vi "fly.vi"(8 "error in (no error)":errorcluster, 11 "FlyWithWings in":refnum<class "FlyWithWings.lvclass">) -> (0 "error out":errorcluster, 2 "String":string, 3 "FlyWithWings out":refnum<class "FlyWithWings.lvclass">)   [LabVIEW 2013, in "FlyWithWings.lvclass"]
uses:
  FlyWithWings.lvclass
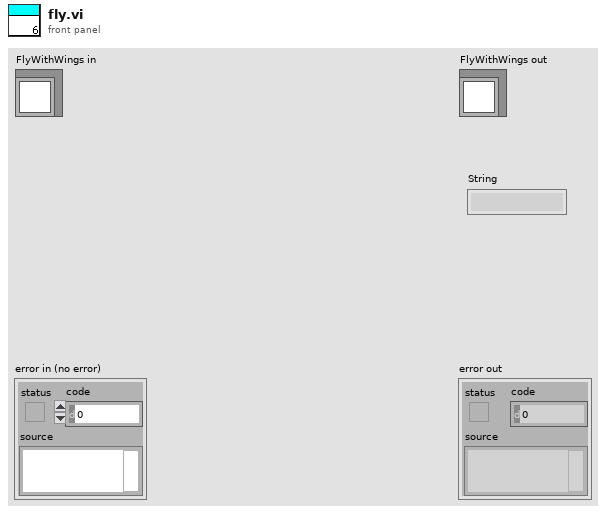
[diagram p1: front panel]
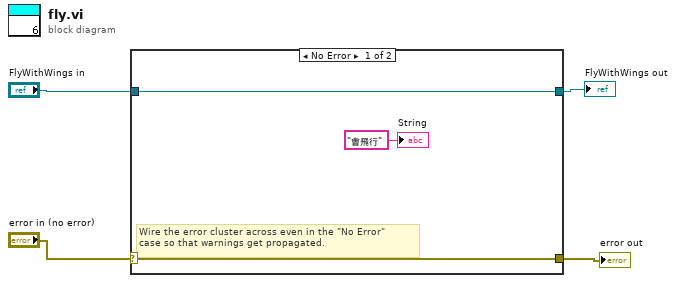
[diagram p0: block diagram]
diagram:
  n1 = case shown="No Error" "error in (no error)" {
    selector: "error in (no error)" -> [w6 w9]
    tunnel: [w6 w9] -> w2
    tunnel: [w7 w8] -> w3
    tunnel: "FlyWithWings in" -> [w7 w8]
    frame No Error {
      # "Wire the error cluster across even in the \"No Error\"\ncase so that warnings get propagated."
      "String" <- "會飛行" ("String")
    }
    frame Error {
    }
  }
  "error out" <- w2
  "FlyWithWings out" <- w3
